vi "SetSettings.vi"(8 "error in (no error)":errorcluster, 10 "Variant":variant, 11 "NHRDCPower in":refnum<class "NHRDCPower.lvclass">) -> (0 "error out":errorcluster, 3 "NHRDCPower Out":refnum<class "NHRDCPower.lvclass">)   [LabVIEW 2018, in "AcPwrPlugins.lvlib" / "NHRDCPower.lvclass"]
doc: "This VI sets the configuration settings, measurement settings, and measurement refresh time."
uses:
  NHRDCPower.lvclass
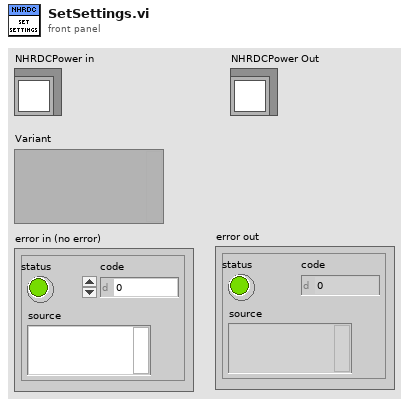
[diagram p1: front panel]
types:
  T1 = typedef "AcPwrPlugins.lvlib/NHRDCPower.lvclass/Device(s)Settings.ctl" = cluster{"MeasName":string, "Modules":T2}
  T2 = typedef "AcPwrPlugins.lvlib/NHRDCPower.lvclass/Modules.ctl" = cluster{"Handle":string, "Name":string, "id query (Yes)":bool, "reset device (Yes)":bool, "Connected":bool, "Initial Battery Detect Voltage (0)":dbl, "SafetySettings":cluster{"SetWatchDog?":bool, "Voltage (V)":dbl, "Current (A)":dbl, "Power (W)":dbl, "Voltage Delay (s)":dbl, "Current Delay (s)":dbl, "Power Delay (s)":dbl}, "Options String":string, "Aperture Time (s)":dbl, "operating state (Off)":i32, "OutputSettings":cluster{"Voltage (V)":dbl, "Current (A)":dbl, "Resistance (Ohms)":dbl, "Power (W)":dbl, "Enable Voltage":bool, "Enable Current":bool, "Enable Resistance":bool, "Enable Power":bool, "Macro After Step Delay  (s)":dbl, "Wait Value (V, A, W)":dbl, "Enable Wait":bool, "Wait on Value":i32}, "SlewRate":cluster{"Set Voltage Rate V/S":dbl, "Set Current Rate A/S":dbl, "Set Resistance Rate R/S":dbl, "Set Power Rate W/S":dbl}, "Macro":cluster{"Save Macro?":bool, "Load Macro From File?":bool, "Run Macro Continuously?":bool, "Use Macros?":bool, "Load Macro File Path":path, "Save Macro File Path":string}, "Regulation Gain (1=100%)":dbl, "UpdatingOntheFly":bool}[]
  T3 = typedef "AcPwrPlugins.lvlib/NHRDCPower.lvclass/Measurements.ctl" = cluster{"Handle":string, "Name":string, "Enabled":bool, "Measurement Value":sgl, "Measurement Type":enum16{"Power", "Current", "Voltage"}}[]
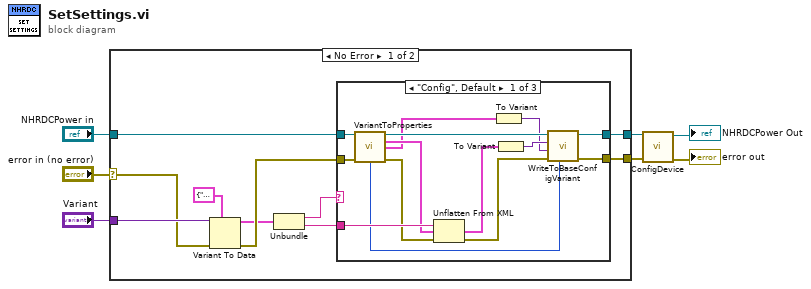
[diagram p0: block diagram]
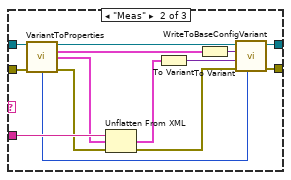
[diagram p2: hidden frame]
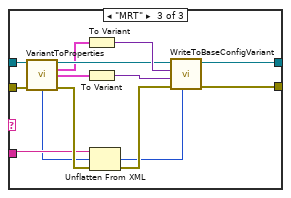
[diagram p3: hidden frame]
diagram:
  n1 = case shown="No Error" "error in (no error)" {
    selector: "error in (no error)" -> [w13 w61]
    tunnel: [w16 w61] -> w4
    tunnel: "NHRDCPower in" -> [w17 w60]
    tunnel: "Variant" -> [w14 _]
    tunnel: [w15 w60] -> w3
    frame No Error {
      n2 = Variant To Data(error in=w13, type=cluster{string, string} {"", ""}, Variant=w14) -> (data=w10:cluster{string, string}, error out=w11:errorcluster)
      n3 = Unbundle(w10) -> (w8:string, w9:string)
      n4 = case shown="\"Config\", Default" w8 {
        tunnel: [w23 w39 w54] -> w16
        tunnel: w17 -> [w30 w44 w59]
        tunnel: [w22 w38 w53] -> w15
        tunnel: w11 -> [w29 w43 w58]
        tunnel: w9 -> [w31 w45 w48]
        frame "Config", Default {
          n5 = call "VariantToProperties.vi"("NHRDCPower in"=w30, "error in (no error)"=w29) -> ("NHRDCPower out"=w21:refnum<class "NHRDCPower.lvclass">, "NHRDC"=w27:T1, "Meas"=w19:T3, "Measurement Refresh Time (ms)"=w20:u32, "error out"=w28:errorcluster)  [unwired: 7 in, 2 out]
          n6 = Unflatten From XML(xml string=w31, type=w27, error in (no error)=w28) -> (value=w26:T1, error out=w24:errorcluster)
          n7 = To Variant(anything=w19) -> (Variant=w18:variant)
          n8 = To Variant(anything=w26) -> (Variant=w25:variant)
          n9 = call "WriteToBaseConfigVariant.vi"("Measurement Refresh Time (ms)"=w20, "error in (no error)"=w24, "Meas"=w18, "Config"=w25, "NHRDCPower in"=w21) -> ("error out"=w23:errorcluster, "NHRDCPower out"=w22:refnum<class "NHRDCPower.lvclass">)  [unwired: 5 in]
        }
        frame "Meas" {
          n10 = call "VariantToProperties.vi"("NHRDCPower in"=w44, "error in (no error)"=w43) -> ("NHRDCPower out"=w37:refnum<class "NHRDCPower.lvclass">, "NHRDC"=w34:T1, "Meas"=w33:T3, "Measurement Refresh Time (ms)"=w36:u32, "error out"=w42:errorcluster)  [unwired: 7 in, 2 out]
          n11 = Unflatten From XML(xml string=w45, type=w33, error in (no error)=w42) -> (value=w32:T3, error out=w40:errorcluster)
          n12 = To Variant(anything=w32) -> (Variant=w35:variant)
          n13 = To Variant(anything=w34) -> (Variant=w41:variant)
          n14 = call "WriteToBaseConfigVariant.vi"("Measurement Refresh Time (ms)"=w36, "error in (no error)"=w40, "Meas"=w35, "Config"=w41, "NHRDCPower in"=w37) -> ("error out"=w39:errorcluster, "NHRDCPower out"=w38:refnum<class "NHRDCPower.lvclass">)  [unwired: 5 in]
        }
        frame "MRT" {
          n15 = call "VariantToProperties.vi"("NHRDCPower in"=w59, "error in (no error)"=w58) -> ("NHRDCPower out"=w52:refnum<class "NHRDCPower.lvclass">, "NHRDC"=w49:T1, "Meas"=w51:T3, "Measurement Refresh Time (ms)"=w47:u32, "error out"=w57:errorcluster)  [unwired: 7 in, 2 out]
          n16 = To Variant(anything=w49) -> (Variant=w56:variant)
          n17 = To Variant(anything=w51) -> (Variant=w50:variant)
          n18 = Unflatten From XML(xml string=w48, type=w47, error in (no error)=w57) -> (value=w46:u32, error out=w55:errorcluster)
          n19 = call "WriteToBaseConfigVariant.vi"("Measurement Refresh Time (ms)"=w46, "error in (no error)"=w55, "Meas"=w50, "Config"=w56, "NHRDCPower in"=w52) -> ("error out"=w54:errorcluster, "NHRDCPower out"=w53:refnum<class "NHRDCPower.lvclass">)  [unwired: 5 in]
        }
      }
    }
    frame Error {
    }
  }
  n20 = call-dynamic "ConfigDevice.vi"("error in (no error)"=w4, "NHRDCPower in"=w3) -> ("error out"=→"error out":errorcluster, "NHRDCPower out"=→"NHRDCPower Out":refnum<class "NHRDCPower.lvclass">)  [unwired: 8 in]
